vi "GetPowerReadings.vi"(4 "error in":errorcluster, 6 "Device Key In":string, 7 "PM Cmds In":refnum<k24>) -> (0 "error out":errorcluster, 1 "Power Readings":string[](array[string]), 2 "Device Key Out":string, 3 "PM Cmds Out":refnum<k24>)   [LabVIEW 2025]
uses:
  C:/Users/20201794/OneDrive - TU Eindhoven/[3] PhD/[4] Scripts/LabVIEW-Samples-v3-0-4/LabVIEW 2010/PowerMeterCommands.dll
  PowerMeterCommands.dll
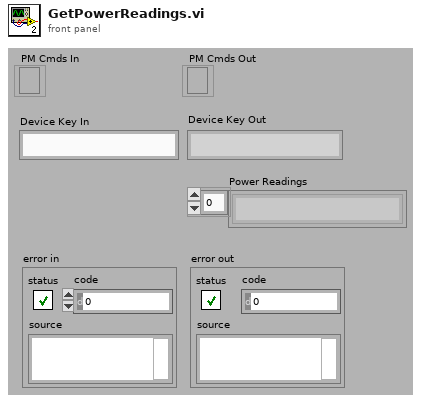
[diagram p1: front panel]
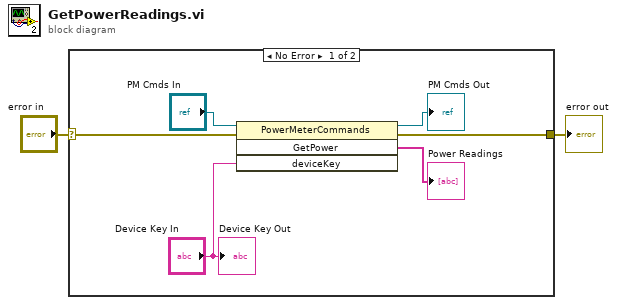
[diagram p0: block diagram]
diagram:
  n1 = case shown="No Error" "error in" {
    selector: "error in" -> [w5 w9]
    tunnel: [w8 w9] -> w2
    frame No Error {
      n2 = invoke class="PowerMeterCommands" method="GetPower"(reference="PM Cmds In", error in=w5, "deviceKey"="Device Key In") -> (reference out=→"PM Cmds Out":refnum<k24>, error out=w8:errorcluster, "GetPower"=→"Power Readings":string[])  [unwired: 1 in, 1 out]
      "Device Key Out" <- "Device Key In"
    }
    frame Error {
    }
  }
  "error out" <- w2
